vi "Launch Nested UIA.vi"(8 "error in (no error)":errorcluster, 9 "Name":string, 10 "UI_Actor":refnum<class "UI_Actor.lvclass">, 11 "Caller UIA in":refnum<class "UI_Actor.lvclass">) -> (0 "error out":errorcluster, 2 "Nested Actor's Enqueuer":refnum<class "Message Enqueuer.lvclass">, 3 "Caller UIA out":refnum<class "UI_Actor.lvclass">)   [LabVIEW 2020, in "UI_Actor.lvlib" / "UI_Actor.lvclass"]
doc: "Lance un UIA en tant que nested.\nName est facultatif mais permet d'identifier l'acteur, principalement dans les remontées d'erreurs."
uses:
  UI_Actor.lvclass
  support/Actor Framework.lvlibp/1abvi3w/vi.lib/ActorFramework/Message Enqueuer/Message Enqueuer.lvclass
  UI_Actor.lvclass/UI_Actor.ctl
  support/Actor Framework.lvlibp/1abvi3w/vi.lib/ActorFramework/Actor/Actor.lvclass
  D:/Projets/STEP AT/UI Actor/support/Actor Framework.lvlibp/1abvi3w/vi.lib/ActorFramework/Actor/Actor.lvclass
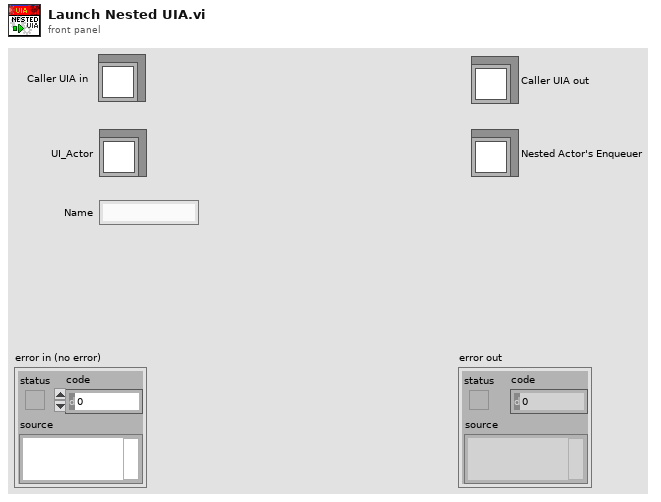
[diagram p1: front panel]
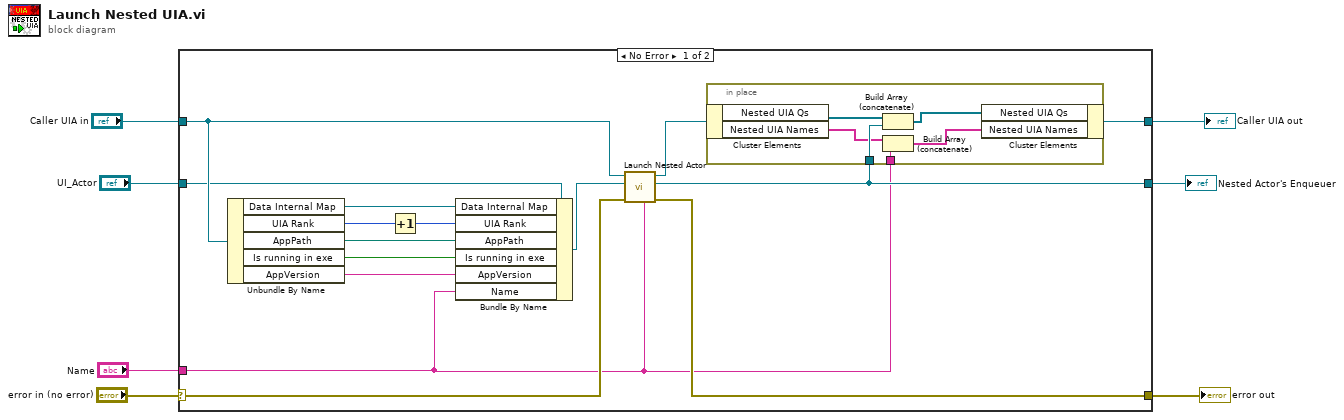
[diagram p0: block diagram]
diagram:
  n1 = case shown="No Error" "error in (no error)" {
    selector: "error in (no error)" -> [w22 w30]
    tunnel: [w21 w30] -> w6
    tunnel: [w11 w29] -> w4
    tunnel: "Caller UIA in" -> [w20 w29]
    tunnel: "UI_Actor" -> [w19 _]
    tunnel: [w12 _] -> w2
    tunnel: "Name" -> [w9 _]
    frame No Error {
      n2 = Unbundle By Name(w20) -> ("Data Internal Map"=w8:refnum<data-value>, "UIA Rank"=w16:i32, "AppPath"=w15:path, "Is running in exe"=w14:bool, "AppVersion"=w10:string)
      n3 = Increment(x=w16) -> (x+1=w17:i32)
      n4 = Bundle By Name(cluster=w19, "Data Internal Map"=w8, "UIA Rank"=w17, "AppPath"=w15, "Is running in exe"=w14, "AppVersion"=w10, "Name"=w9) -> (w18:refnum<class "UI_Actor.lvclass">)
      n5 = call "Launch Nested Actor.vi"("Debug Alias"=w9, "error in (no error)"=w22, "Nested Actor"=w18, "Caller Actor in"=w20) -> ("error out"=w21:errorcluster, "Nested Actor's Enqueuer"=w12:refnum<class "Message Enqueuer.lvclass">, "Caller Actor out"=w13:refnum<class "UI_Actor.lvclass">)  [unwired: 5 in]
      n6 = in-place {
        in-place-border: w12 -> [w26]
        in-place-border: w9 -> [w23]
        n7 = in-place-cluster #1(w13) -> ("Nested UIA Qs"=w28:refnum<class "Message Enqueuer.lvclass">[], "Nested UIA Names"=w25:string[])
        n8 = Build Array (concatenate)(w28, w26) -> (w27:refnum<class "Message Enqueuer.lvclass">[])
        n9 = Build Array (concatenate)(w25, w23) -> (w24:string[])
        n10 = in-place-cluster #1("Nested UIA Qs"=w27, "Nested UIA Names"=w24) -> (w11:refnum<class "UI_Actor.lvclass">)
      }
    }
    frame Error {
    }
  }
  "error out" <- w6
  "Caller UIA out" <- w4
  "Nested Actor's Enqueuer" <- w2
